vi "Mysql data reader 1D double.vi"(8 "error in (no error)":errorcluster, 11 ".NET Refnum in":refnum<k24>) -> (0 "error out":errorcluster, 3 "Array":dbl[](array[numeric]))   [LabVIEW 2020, in "mysql.lvlib" / "mysql.lvclass"]
uses:
  mysql.lvclass
  MySql.Data
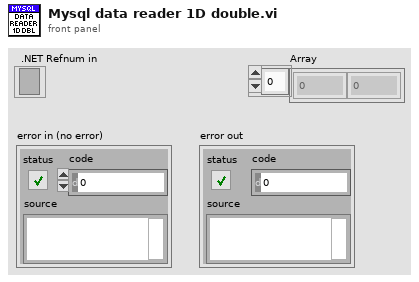
[diagram p1: front panel]
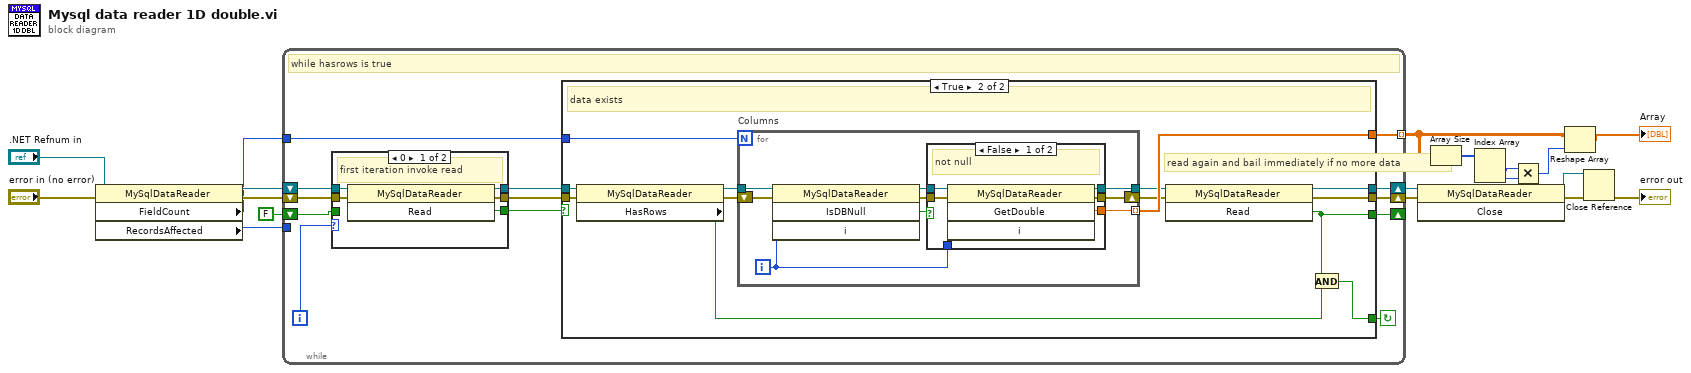
[diagram p0: block diagram]
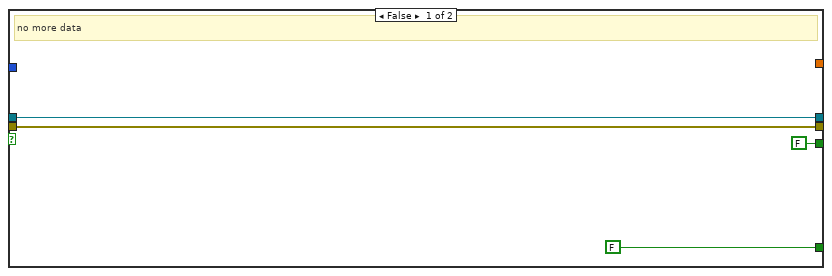
[diagram p3: hidden frame]
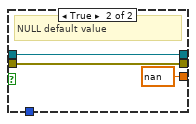
[diagram p4: hidden frame]
diagram:
  n1 = property class="MySqlDataReader"(reference=".NET Refnum in", error in="error in (no error)") -> (reference out=w13:refnum<k24>, error out=w12:errorcluster, "FieldCount"=w10:i32, "RecordsAffected"=w18:i32)
  n2 = while {
    tunnel: w10 -> [w31]
    tunnel: [w30] -> w5 mode=indexing
    shift-right: [w28] -> w15
    shift-left: w12 -> [w25]
    shift-right: [w29] -> w14
    shift-left: w13 -> [w26]
    tunnel: w18 -> [_]
    shift-right: [w20] -> _
    shift-left: FALSE ("Read") -> [w19]
    i -> [w24]
    stop <- w27 continue-if-true
    # "while hasrows is true"
    n3 = case shown="0" w24 {
      tunnel: w25 -> [w36 w38]
      tunnel: [w35 w38] -> w23
      tunnel: w26 -> [w34 w39]
      tunnel: [w33 w39] -> w22
      tunnel: [w32 w37] -> w21
      tunnel: w19 -> [_ w37]
      frame 0 {
        # "first iteration invoke read"
        n4 = invoke class="MySqlDataReader" method="Read"(reference=w34, error in=w36) -> (reference out=w33:refnum<k24>, error out=w35:errorcluster, "Read"=w32:bool)  [unwired: 1 in]
      }
      frame 1.., Default {
        # "read after for other iterations"
      }
    }
    n5 = case shown="True" w21 {
      tunnel: w31 -> [_ w56]
      tunnel: [_ w55] -> w30
      tunnel: w23 -> [w42 w54]
      tunnel: w22 -> [w43 w53]
      tunnel: [w43 w48] -> w29
      tunnel: [w42 w49] -> w28
      tunnel: [FALSE ("HasRows") w45] -> w27
      tunnel: [FALSE ("Read") w44] -> w20
      frame False {
        # "no more data"
      }
      frame True {
        # "read again and bail immediately if no more data"
        # "data exists"
        n6 = property class="MySqlDataReader"(reference=w53, error in=w54) -> (reference out=w52:refnum<k24>, error out=w51:errorcluster, "HasRows"=w46:bool)
        n7 = for "Columns" {
          N: w56 -> [_]
          tunnel: w52 -> [w60]
          shift-right: [w65] -> w50
          shift-left: w51 -> [w61]
          tunnel: [w64] -> w55 mode=indexing
          tunnel: [w63] -> w47
          i -> [w62]
          n8 = invoke class="MySqlDataReader" method="IsDBNull"(reference=w60, error in=w61, "i"=w62) -> (reference out=w59:refnum<k24>, error out=w58:errorcluster, "IsDBNull"=w57:bool)  [unwired: 1 in, 1 out]
          n9 = case shown="False" w57 {
            tunnel: [w71 w73] -> w65
            tunnel: [w70 nan ("GetDouble")] -> w64
            tunnel: [w69 w74] -> w63
            tunnel: w62 -> [w68 _]
            tunnel: w59 -> [w67 w74]
            tunnel: w58 -> [w66 w73]
            frame False {
              # "not null"
              n10 = invoke class="MySqlDataReader" method="GetDouble"(reference=w67, error in=w66, "i"=w68) -> (reference out=w69:refnum<k24>, error out=w71:errorcluster, "GetDouble"=w70:dbl)  [unwired: 1 in, 1 out]
            }
            frame True {
              # "NULL default value"
            }
          }
        }
        n11 = invoke class="MySqlDataReader" method="Read"(reference=w47, error in=w50) -> (reference out=w48:refnum<k24>, error out=w49:errorcluster, "Read"=w44:bool)  [unwired: 1 in]
        n12 = And(x=w44, y=w46) -> (x .and. y?=w45:bool)
      }
    }
  }
  n13 = invoke class="MySqlDataReader" method="Close"(reference=w14, error in=w15) -> (reference out=w17:refnum<k24>, error out=w16:errorcluster)  [unwired: 1 in, 1 out]
  n14 = Array Size(array=w5) -> (size(s)=w4:i32[])
  n15 = Index Array(array=w4) -> (element #1=w3:i32, element #2=w2:i32)  [unwired: 2 in]
  n16 = Multiply(x=w3, y=w2) -> (x*y=w1:i32)
  n17 = Reshape Array(w5, w1) -> (→"Array":dbl[])
  n18 = Close Reference(reference=w17, error in (no error)=w16) -> (error out=→"error out":errorcluster)
